vi "CODMn启动命令 (子VI).vi"(9 "强制切换":bool, 10 "CODMn量程切换":enum32{"H", "L", "AUTO"}(ring)=enum."AUTO", 11 "启动测量模式":T1) -> (0 "错误输出":errorcluster)   [LabVIEW 2016, in "质控单元.lvlib"]
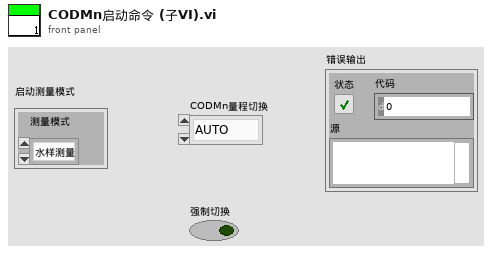
[diagram p1: front panel]
types:
  T1 = cluster{"测量模式":enum16{"水样测量", "标样核查", "零点核查", "跨度核查", "空白测试", "加标回收", "平行样", "校零", "校标"}}
  T2 = cluster{"命令":string, "测量模式":enum16{"水样测量", "标样核查", "零点核查", "跨度核查", "空白测试", "加标回收", "平行样", "校零", "校标"}, "CODMn量程切换":enum32{"H", "L", "AUTO"}}
  T3 = enum16{"水样测量", "标样核查", "零点核查", "跨度核查", "空白测试", "加标回收", "平行样", "校零", "校标"}
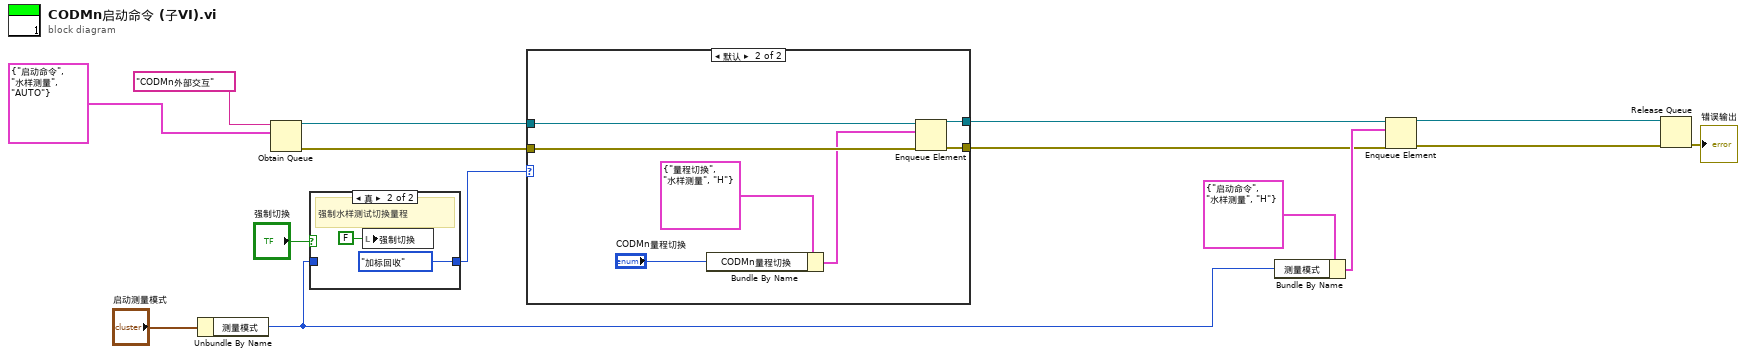
[diagram p0: block diagram]
diagram:
  n1 = Unbundle By Name("启动测量模式") -> ("测量模式"=w3:T3)
  n2 = Obtain Queue(name (unnamed)="CODMn外部交互" ("名称（未命名）"), element data type=T2 {"命令"="启动命令", "测量模式"=enum."水样测量", "CODMn量程切换"=enum."AUTO"} ("元素")) -> (queue out=w8:refnum<queue>, error out=w7:errorcluster)  [unwired: 3 in, 1 out]
  n3 = case shown="真" "强制切换" {
    tunnel: w3 -> [w16 _]
    tunnel: [w16 T3."加标回收" ("测量模式")] -> w2
    frame False {
    }
    frame True {
      # "强制水样测试切换量程"
      n4 = local write "强制切换"(FALSE ("强制切换")) -> ()
    }
  }
  n5 = case shown="默认" w2 {
    tunnel: w8 -> [w20 w27]
    tunnel: w7 -> [w19 w26]
    tunnel: [w20 w25] -> w6
    tunnel: [w19 w24] -> w5
    frame "水样测量" {
    }
    frame Default {
      n6 = Bundle By Name(cluster=T2 {"命令"="量程切换", "测量模式"=enum."水样测量", "CODMn量程切换"=enum."H"} ("元素"), "CODMn量程切换"="CODMn量程切换") -> (w22:T2)
      n7 = Enqueue Element(queue=w27, element=w22, error in (no error)=w26) -> (queue out=w25:refnum<queue>, error out=w24:errorcluster)  [unwired: 1 in, 1 out]
    }
  }
  n8 = Bundle By Name(cluster=T2 {"命令"="启动命令", "测量模式"=enum."水样测量", "CODMn量程切换"=enum."H"} ("元素"), "测量模式"=w3) -> (w9:T2)
  n9 = Enqueue Element(queue=w6, element=w9, error in (no error)=w5) -> (queue out=w13:refnum<queue>, error out=w12:errorcluster)  [unwired: 1 in, 1 out]
  n10 = Release Queue(queue=w13, error in (no error)=w12) -> (error out=→"错误输出":errorcluster)  [unwired: 1 in, 2 out]
